vi "XNET CAN Frame to NI-CAN Table.vi"(7 "Hexadecimal?":bool, 10 "CAN Frames (from XNET Read)":T1[](array[typedef]) {"payload" format="%x"; "timestamp" format="%<%.7X\n%x>T"; "type" items=["CAN Data"=0, "CAN Remote"=1, "Delay"=224]; "identifier" format="%x"}) -> (3 "Output Array":string[][](array[string]))   [LabVIEW 2010, in "CAN Log Transfer and Convert.lvlib"]
uses:
  <vilib>/xnet/xnet.llb/XNET Frame CAN.ctl
  <vilib>/xnet/xnet.llb/XNET Frame Type CAN.ctl
  CAN Log Transfer and Convert.lvlib
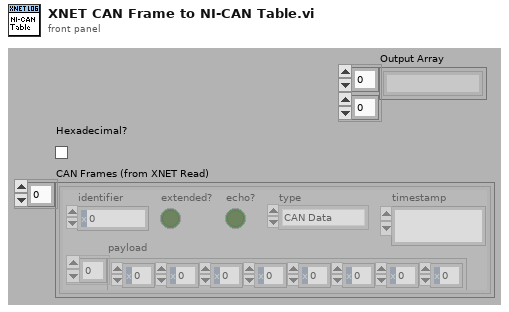
[diagram p1: front panel]
types:
  T1 = typedef "XNET Frame CAN.ctl" = cluster{"timestamp":timestamp, "payload":u8[], "identifier":u32, "type":T2, "extended?":bool, "echo?":bool}
  T2 = typedef "XNET Frame Type CAN.ctl" = u8
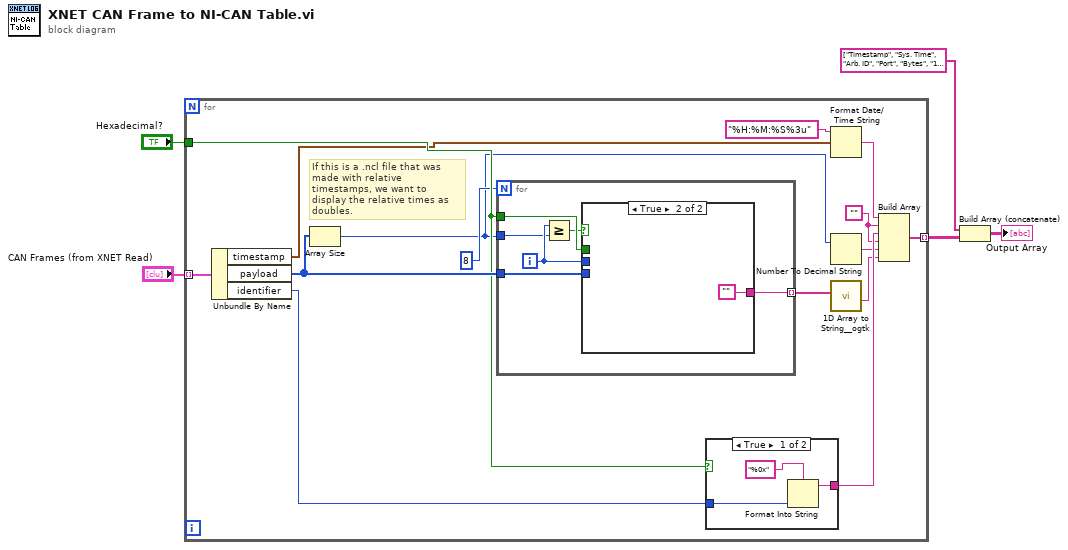
[diagram p0: block diagram]
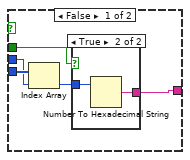
[diagram p2: hidden frame]
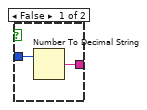
[diagram p3: hidden frame]
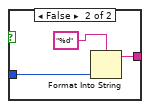
[diagram p4: hidden frame]
diagram:
  n1 = for {
    tunnel: "CAN Frames (from XNET Read)" -> [w20] mode=indexing
    tunnel: "Hexadecimal?" -> [w17]
    tunnel: [w16] -> w3 mode=indexing
    w6 = ""
    # "If this is a .ncl file that was made with relative timestamps, we want to display the relative times as doubles."
    n2 = Unbundle By Name(w20) -> ("timestamp"=w15:timestamp, "payload"=w18:u8[], "identifier"=w19:u32)
    n3 = Array Size(array=w18) -> (size(s)=w9:i32)
    n4 = for {
      N: 8 -> [_]
      tunnel: w18 -> [w24]
      tunnel: [w26] -> w10 mode=indexing
      tunnel: w17 -> [w25]
      tunnel: w9 -> [w22]
      i -> [w23]
      n5 = Greater Or Equal?(x=w23, y=w22) -> (x >= y?=w21:bool)
      n6 = case shown="True" w21 {
        tunnel: [w31 ""] -> w26
        tunnel: w25 -> [w30 _]
        tunnel: w24 -> [w29 _]
        tunnel: w23 -> [w28 _]
        frame False {
          n7 = Index Array(array=w29, index=w28) -> (element=w27:u8)
          n8 = case shown="True" w30 {
            tunnel: [w33 w35] -> w31
            tunnel: w27 -> [w32 w34]
            frame False {
              n9 = Number To Decimal String(number=w32) -> (decimal integer string=w33:string)  [unwired: 1 in]
            }
            frame True {
              n10 = Number To Hexadecimal String(2:w34) -> (0:w35:string)  [unwired: 1 in]
            }
          }
        }
        frame True {
        }
      }
    }
    n11 = case shown="True" w17 {
      tunnel: w19 -> [w38 w41]
      tunnel: [w37 w40] -> w13
      frame True {
        n12 = Format Into String(format string="%0x", w38) -> (resulting string=w37:string)  [unwired: 2 in, 1 out]
      }
      frame False {
        n13 = Format Into String(format string="%d", w41) -> (resulting string=w40:string)  [unwired: 2 in, 1 out]
      }
    }
    n14 = Format Date/Time String(time format string (%c)="%H:%M:%S%3u", seconds (now)=w15) -> (date/time string=w14:string)  [unwired: 1 in]
    n15 = Number To Decimal String(number=w9) -> (decimal integer string=w12:string)  [unwired: 1 in]
    n16 = call <userlib>:"1D Array to String__ogtk.vi"("Array of Strings"=w10) -> ("delimited string"=w8:string)  [unwired: 10 in]
    n17 = Build Array(w14, w6, w13, w6, w12, w8) -> (w16:string[])
  }
  n18 = Build Array (concatenate)(string[] ["Timestamp", "Sys. Time", "Arb. ID", "Port", "Bytes", "1", "2", "3", "4", "5", "6", "7", "8"], w3) -> (→"Output Array":string[][])
